vi "roboRIO v1.0 Shutdown DIO.vi"(8 "error in (no error)":errorcluster, 10 "Channel List":T3, 11 "myRIO Ref In":T1) -> (0 "error out":errorcluster, 3 "myRIO Ref Out":T1)   [LabVIEW 2021]
uses:
  <vilib>/myRIO/Common/Instrument Driver Framework/myRIO v1.0/DIO/typedefs/DIO Channels List.ctl
  <vilib>/myRIO/Common/Instrument Driver Framework/myRIO v1.0/DIO/typedefs/DIO Channels Enum.ctl
  <vilib>/myRIO/Common/Instrument Driver Framework/Utilities/typedefs/myRIO v1.0 Reference.ctl
  <vilib>/myRIO/Common/Instrument Driver Framework/Utilities/typedefs/Generic FPGA Reference.ctl
  <vilib>/myRIO/Common/Instrument Driver Framework/roboRIO v1.0/DIO/typedefs/roboRIO DIO FPGA Reference.ctl
  <vilib>/myRIO/Common/Instrument Driver Framework/roboRIO v1.0/DIO/typedefs/roboRIO DIO Bank Enum.ctl
  <vilib>/Utility/error.llb/Error Cluster From Error Code.vi
  <vilib>/rvi/errors/niLvFpgaAdjustHostInterfaceError.vi
  <vilib>/rvi/interface/nirviReadWriteControl/nirviReadWriteControl.xnode
  NiFpgaLv.dll
  <vilib>/rvi/interface/Simulation/niFpgaSimulationCallBeginRW.vi
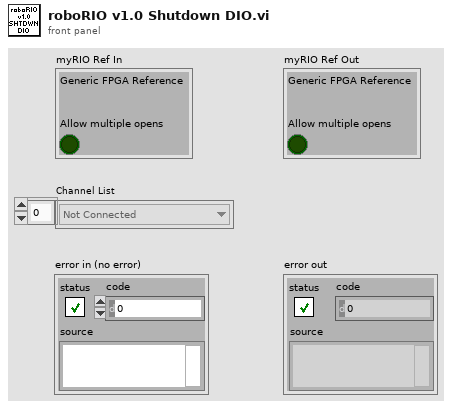
[diagram p1: front panel]
types:
  T1 = typedef "myRIO v1.0 Reference.ctl" = cluster{"Generic FPGA Reference":T2, "Allow multiple opens":bool}
  T2 = typedef "Generic FPGA Reference.ctl" = refnum<k20>
  T3 = typedef "DIO Channels List.ctl" = T4[]
  T4 = typedef "DIO Channels Enum.ctl" = enum16{"Not Connected", "C/DIO0", "C/DIO1", "C/DIO2", "C/DIO3", "C/DIO4", "C/DIO5", "C/DIO6", "C/DIO7", "A/DIO0", "A/DIO1", "A/DIO2", "A/DIO3", "A/DIO4", "A/DIO5", "A/DIO6", "A/DIO7", "A/DIO8", "A/DIO9", "A/DIO10", "A/DIO11", "A/DIO12", "A/DIO13", "A/DIO14", "A/DIO15", "A/DIO16", "A/DIO17", "A/DIO18", "A/DIO19", "B/DIO0", "B/DIO1", "B/DIO2", "B/DIO3", "B/DIO4", "B/DIO5", "B/DIO6", "B/DIO7", "B/DIO8", "B/DIO9", "B/DIO10", "B/DIO11", "B/DIO12", "B/DIO13", "B/DIO14", "B/DIO15", "B/DIO16", "B/DIO17", "B/DIO18", "B/DIO19", "LED0", "LED1", "LED2", "LED3", "Button0", "DIO/DIO0", "DIO/DIO1", "DIO/DIO2", "DIO/DIO3", "DIO/DIO4", "DIO/DIO5", "DIO/DIO6", "DIO/DIO7", "DIO/DIO8", "DIO/DIO9", "SPI/CS0", "SPI/CS1", "SPI/CS2", "SPI/CS3", "LED RADIO (Green)", "LED RADIO (Red)", "LED COMM (Green)", "LED COMM (Red)", "LED MODE (Green)", "LED MODE (Red)"}
  T5 = typedef "roboRIO DIO Bank Enum.ctl" = enum32{"None", "B/DIO7:0", "B/DIO15:8", "DIO/DIO7:0", "DIO/DIO9:8", "SPI/CS3:0", "LED", "Button0"}
  T6 = typedef "roboRIO DIO FPGA Reference.ctl" = refnum<k20>
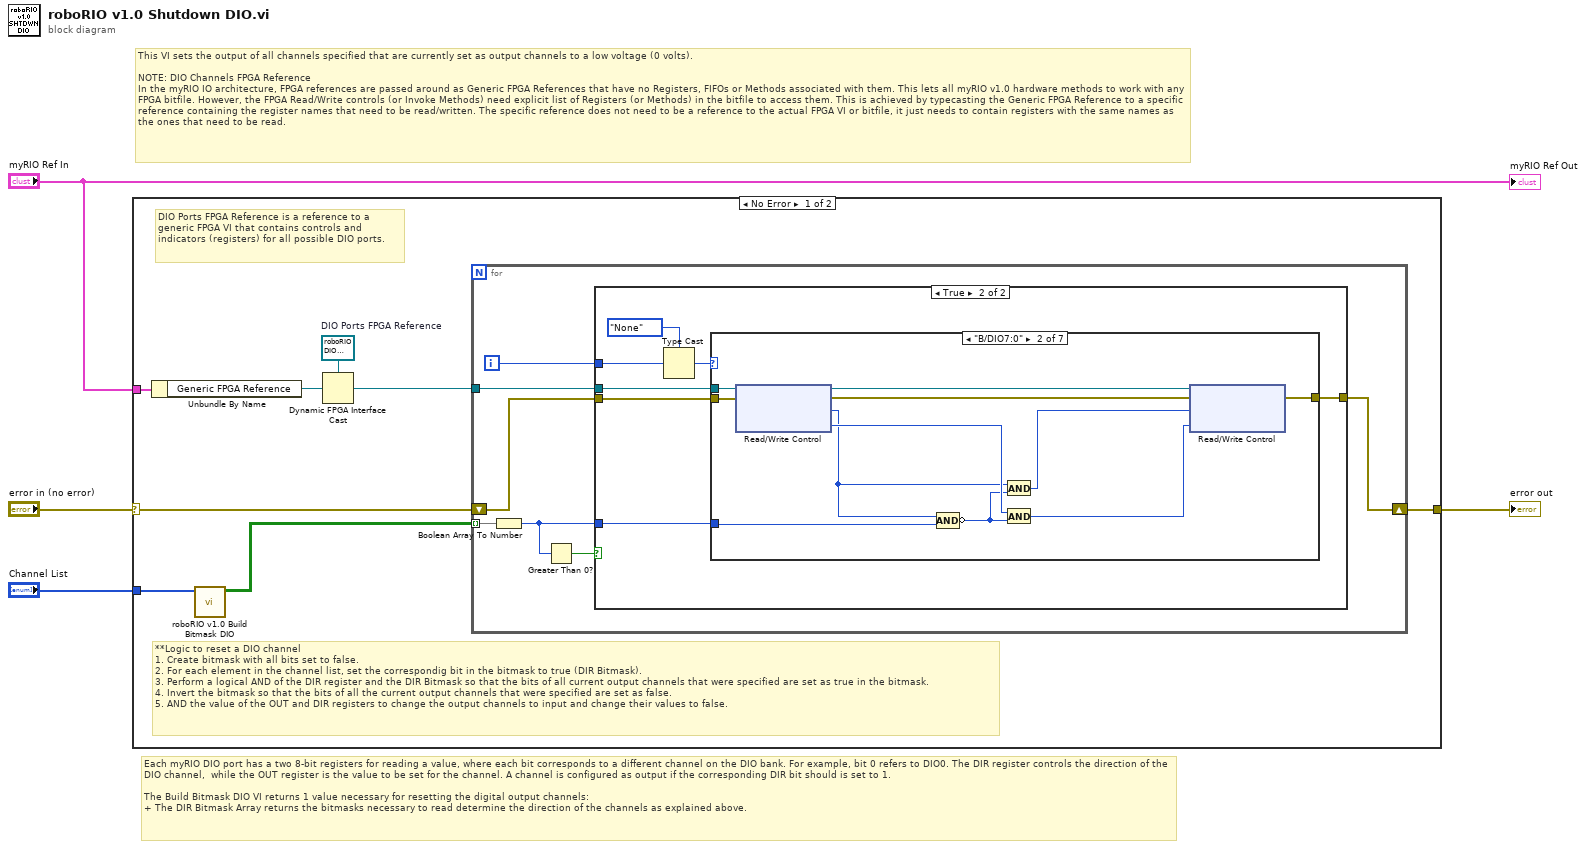
[diagram p0: block diagram]
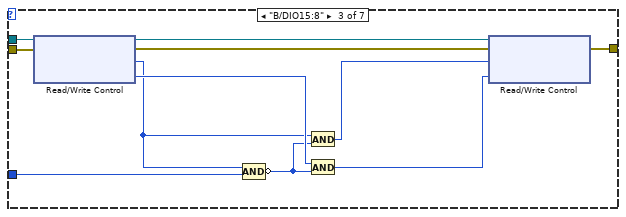
[diagram p4: hidden frame]
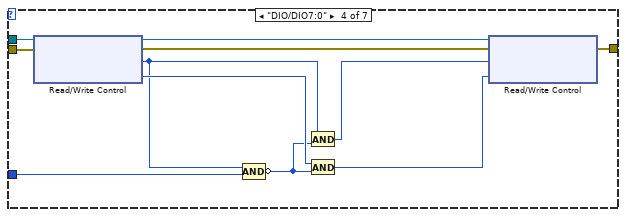
[diagram p5: hidden frame]
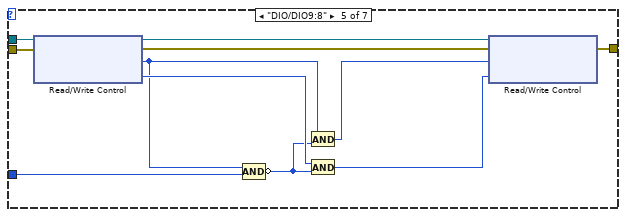
[diagram p6: hidden frame]
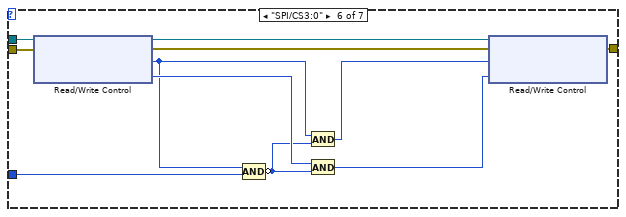
[diagram p7: hidden frame]
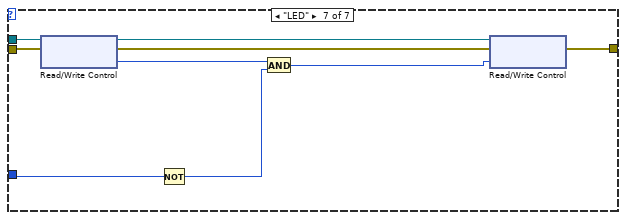
[diagram p8: hidden frame]
diagram:
  # "Each myRIO DIO port has a two 8-bit registers for reading a value, where each bit corresponds to a different channel on the DIO bank. For example, bit 0 refers to DIO0. The DIR register controls the direction of the DIO channel,  while the OUT register is the value to be set for the channel. A channel is configured as output if the corresponding DIR bit should is set to 1.\n\nThe Build Bitmask DIO VI returns 1 value necessary for resetting the digital output channels:\n+ The DIR Bitmask Array returns the bitmasks necessary to read determine the direction of the channels as explained above."
  # "This VI sets the output of all channels specified that are currently set as output channels to a low voltage (0 volts).\n\nNOTE: DIO Channels FPGA Reference\nIn the myRIO IO architecture, FPGA references are passed around as Generic FPGA References that have no Registers, FIFOs or Methods associated with them. This lets all myRIO v1.0 hardware methods to work with any FPGA bitfile. However, the FPGA Read/Write controls (or Invoke Methods) need explicit list of Registers (or Methods) in the bitfile to access them. This is achieved by typecasting the Generic FPGA Reference to a specific reference containing the register names that need to be read/written. The specific reference does not need to be a reference to the actual FPGA VI or bitfile, it just needs to contain registers with the same names as the ones that need to be read."
  n1 = case shown="No Error" "error in (no error)" {
    selector: "error in (no error)" -> [w7 w93]
    tunnel: "myRIO Ref In" -> [w6 _]
    tunnel: [w10 w93] -> w3
    tunnel: "Channel List" -> [w9 _]
    frame No Error {
      w12 = T6 refnum  # DIO Ports FPGA Reference
      # "**Logic to reset a DIO channel\n1. Create bitmask with all bits set to false.\n2. For each element in the channel list, set the correspondig bit in the bitmask to true (DIR Bitmask).\n3. Perform a logical AND of the DIR register and the DIR Bitmask so that the bits of all current output channels that were specified are set as true in the bitmask.\n4. Invert the bitmask so that the bits of all the current output channels that were specified are set as false.\n5. AND the value of the OUT and DIR registers to change the output channels to input and change their values to false."
      # "DIO Ports FPGA Reference is a reference to a generic FPGA VI that contains controls and indicators (registers) for all possible DIO ports."
      n2 = Unbundle By Name(w6) -> ("Generic FPGA Reference"=w5:T2)
      n3 = call <vilib>:"roboRIO v1.0 Build Bitmask DIO.vi"("Channel List"=w9) -> ("DIR Bitmask Array"=w8:bool[][])  [unwired: 8 in, 2 out]
      n4 = Dynamic FPGA Interface Cast(Session In=w12, Type=w5) -> (Session Out=w11:T6)
      n5 = for {
        tunnel: w8 -> [w17] mode=indexing
        tunnel: w11 -> [w19]
        shift-right: [w16] -> w10
        shift-left: w7 -> [w15]
        i -> [w18]
        n6 = Boolean Array To Number(Boolean array=w17) -> (number=w13:u8)
        n7 = Greater Than 0?(x=w13) -> (x > 0?=w14:bool)
        n8 = case shown="True" w14 {
          tunnel: w19 -> [_ w27]
          tunnel: w18 -> [_ w26]
          tunnel: w13 -> [_ w23]
          tunnel: [w20 w22] -> w16
          tunnel: w15 -> [w20 w21]
          frame False {
          }
          frame True {
            n9 = Type Cast(type=roboRIO_DIO_Bank_Enum."None" ("DIO Bank Enum"), x=w26) -> (*(type *) &x=w24:T5)
            n10 = case shown="\"B/DIO7:0\"" w24 {
              tunnel: w27 -> [_ w39 w50 w61 w72 w83 w91]
              tunnel: w23 -> [_ w37 w48 w59 w70 w81 w89]
              tunnel: [w28 w35 w46 w57 w68 w79 w92] -> w22
              tunnel: w21 -> [w28 w34 w45 w56 w67 w78 w90]
              frame "None", Default {
              }
              frame "B/DIO7:0" {
                n11 = xnode "Read/Write Control"("FPGA VI Reference In"=w39, "error in"=w34) -> ("FPGA VI Reference Out"=w38:T6, "error out"=w36:errorcluster, "DIO.B_7:0.DIR"=w31:u8, "DIO.B_7:0.OUT"=w33:u8)
                n12 = Compound Arithmetic op=AND(w31, w37) -> (invert w30:u8)
                n13 = And(x=w31, y=w30) -> (x .and. y?=w29:u8)
                n14 = And(x=w33, y=w30) -> (x .and. y?=w32:u8)
                n15 = xnode "Read/Write Control"("FPGA VI Reference In"=w38, "error in"=w36, "DIO.B_7:0.DIR"=w29, "DIO.B_7:0.OUT"=w32) -> ("error out"=w35:errorcluster)  [unwired: 1 out]
              }
              frame "B/DIO15:8" {
                n16 = xnode "Read/Write Control"("FPGA VI Reference In"=w50, "error in"=w45) -> ("FPGA VI Reference Out"=w49:T6, "error out"=w47:errorcluster, "DIO.B_15:8.DIR"=w41:u8, "DIO.B_15:8.OUT"=w44:u8)
                n17 = Compound Arithmetic op=AND(w41, w48) -> (invert w40:u8)
                n18 = And(x=w41, y=w40) -> (x .and. y?=w42:u8)
                n19 = And(x=w44, y=w40) -> (x .and. y?=w43:u8)
                n20 = xnode "Read/Write Control"("FPGA VI Reference In"=w49, "error in"=w47, "DIO.B_15:8.DIR"=w42, "DIO.B_15:8.OUT"=w43) -> ("error out"=w46:errorcluster)  [unwired: 1 out]
              }
              frame "DIO/DIO7:0" {
                n21 = xnode "Read/Write Control"("FPGA VI Reference In"=w61, "error in"=w56) -> ("FPGA VI Reference Out"=w60:T6, "error out"=w58:errorcluster, "DIO.DIO_7:0.DIR"=w52:u8, "DIO.DIO_7:0.OUT"=w55:u8)
                n22 = Compound Arithmetic op=AND(w52, w59) -> (invert w51:u8)
                n23 = And(x=w52, y=w51) -> (x .and. y?=w53:u8)
                n24 = And(x=w55, y=w51) -> (x .and. y?=w54:u8)
                n25 = xnode "Read/Write Control"("FPGA VI Reference In"=w60, "error in"=w58, "DIO.DIO_7:0.DIR"=w53, "DIO.DIO_7:0.OUT"=w54) -> ("error out"=w57:errorcluster)  [unwired: 1 out]
              }
              frame "DIO/DIO9:8" {
                n26 = xnode "Read/Write Control"("FPGA VI Reference In"=w72, "error in"=w67) -> ("FPGA VI Reference Out"=w71:T6, "error out"=w69:errorcluster, "DIO.DIO_9:8.DIR"=w63:u8, "DIO.DIO_9:8.OUT"=w66:u8)
                n27 = Compound Arithmetic op=AND(w63, w70) -> (invert w62:u8)
                n28 = And(x=w63, y=w62) -> (x .and. y?=w64:u8)
                n29 = And(x=w66, y=w62) -> (x .and. y?=w65:u8)
                n30 = xnode "Read/Write Control"("FPGA VI Reference In"=w71, "error in"=w69, "DIO.DIO_9:8.DIR"=w64, "DIO.DIO_9:8.OUT"=w65) -> ("error out"=w68:errorcluster)  [unwired: 1 out]
              }
              frame "SPI/CS3:0" {
                n31 = xnode "Read/Write Control"("FPGA VI Reference In"=w83, "error in"=w78) -> ("FPGA VI Reference Out"=w82:T6, "error out"=w80:errorcluster, "DIO.SPI_CS3:0.DIR"=w74:u8, "DIO.SPI_CS3:0.OUT"=w77:u8)
                n32 = Compound Arithmetic op=AND(w74, w81) -> (invert w73:u8)
                n33 = And(x=w74, y=w73) -> (x .and. y?=w75:u8)
                n34 = And(x=w77, y=w73) -> (x .and. y?=w76:u8)
                n35 = xnode "Read/Write Control"("FPGA VI Reference In"=w82, "error in"=w80, "DIO.SPI_CS3:0.DIR"=w75, "DIO.SPI_CS3:0.OUT"=w76) -> ("error out"=w79:errorcluster)  [unwired: 1 out]
              }
              frame "LED" {
                n36 = xnode "Read/Write Control"("FPGA VI Reference In"=w91, "error in"=w90) -> ("FPGA VI Reference Out"=w87:T6, "error out"=w86:errorcluster, "DO.LED 5:0"=w85:u8)
                n37 = Not(x=w89) -> (.not. x?=w88:u8)
                n38 = And(x=w85, y=w88) -> (x .and. y?=w84:u8)
                n39 = xnode "Read/Write Control"("FPGA VI Reference In"=w87, "error in"=w86, "DO.LED 5:0"=w84) -> ("error out"=w92:errorcluster)  [unwired: 1 out]
              }
            }
          }
        }
      }
    }
    frame Error {
    }
  }
  "error out" <- w3
  "myRIO Ref Out" <- "myRIO Ref In"
